vi "TblCheck.vi"(4 "error in":errorcluster, 7 "connection reference":T1) -> (0 "error out":errorcluster, 2 "tables":string[](array[string]), 3 "conn ref out":T1)   [LabVIEW 2010]
uses:
  <vilib>/addons/database/Connection.llb/Conn ObjectReference.ctl
  <vilib>/addons/database/NI_Database_API.lvlib
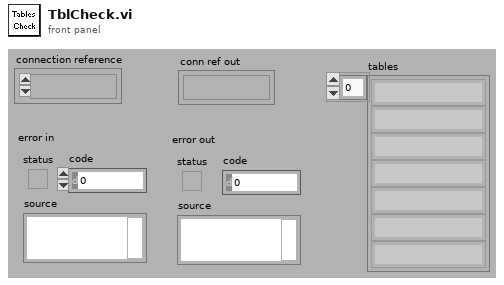
[diagram p1: front panel]
types:
  T1 = typedef "NI_Database_API.lvlib/Conn ObjectReference.ctl" = refnum<k1>
  T2 = cluster{"type":string, "units":string, "n":i32}[]
  T3 = typedef "NI_Database_API.lvlib/DB Tools Column Info.ctl" = cluster{"column name":string, "data type":T4, "size":i32, "allow null?":bool}
  T4 = typedef "NI_Database_API.lvlib/DB Tools DataTypes.ctl" = enum16{"String", "Long (I32)", "Single (SGL)", "Double (DBL)", "Date/Time", "Binary"}
  T5 = cluster{"key":string, "column information":T3[]}[]
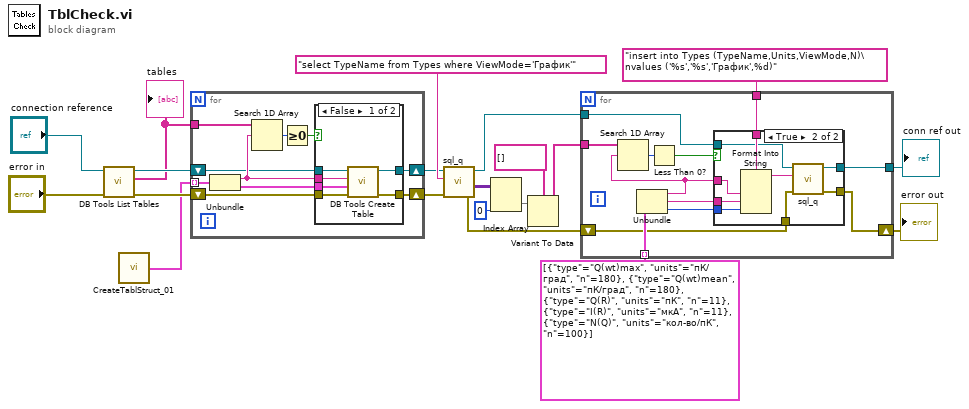
[diagram p0: block diagram]
diagram:
  n1 = call <vilib>:"DB Tools List Tables.vi"("error in (no error)"="error in", "connection reference"="connection reference") -> ("error out"=w19:errorcluster, "tables"=w18:string[], "connection reference out"=w20:T1)  [unwired: 3 in]
  "tables" <- w18
  n2 = call "CreateTablStruct_01.vi"() -> ("Array"=w15:T5)
  n3 = for {
    tunnel: w15 -> [w27] mode=indexing
    tunnel: w18 -> [w30]
    shift-right: [w22] -> w6
    shift-left: w20 -> [w21]
    shift-right: [w24] -> w5
    shift-left: w19 -> [w23]
    n4 = Unbundle(w27) -> ("key"=w26:string, "column information"=w25:T3[])
    n5 = Search 1D Array(1D array=w30, element=w26) -> (index of element=w29:i32)  [unwired: 1 in]
    n6 = Greater Or Equal To 0?(x=w29) -> (x >= 0?=w28:bool)
    n7 = case shown="False" w28 {
      tunnel: w26 -> [w36 _]
      tunnel: w25 -> [w35 _]
      tunnel: [w34 w38] -> w24
      tunnel: w23 -> [w33 w38]
      tunnel: [w32 w37] -> w22
      tunnel: w21 -> [w31 w37]
      frame False {
        n8 = call <vilib>:"DB Tools Create Table.vi"("error in (no error)"=w33, "column information"=w35, "table"=w36, "connection reference"=w31) -> ("error out"=w34:errorcluster, "connection reference out"=w32:T1)  [unwired: 4 in]
      }
      frame True {
      }
    }
  }
  n9 = call "sql_q.vi"("error in"=w5, "SQL query"="select TypeName from Types where ViewMode='График'", "connect ref"=w6) -> ("error out"=w3:errorcluster, "recordset data"=w11:variant[][], "conn ref out"=w4:T1)  [unwired: 1 in, 1 out]
  n10 = Index Array(array=w11, index (col)=0 ("disabled index (col)")) -> (element=w9:variant[])  [unwired: 1 in]
  n11 = Variant To Data(Variant=w9, type=string[] []) -> (data=w7:string[])  [unwired: 1 in, 1 out]
  n12 = for {
    tunnel: "insert into Types (TypeName,Units,ViewMode,N)\nvalues ('%s','%s','График',%d)" -> [w50]
    tunnel: T2 [{"type"="Q(wt)max", "units"="пК/град", "n"=180}, {"type"="Q(wt)mean", "units"="пК/град", "n"=180}, {"type"="Q(R)", "units"="пК", "n"=11}, {"type"="I(R)", "units"="мкА", "n"=11}, {"type"="N(Q)", "units"="кол-во/пК", "n"=100}] -> [w47] mode=indexing
    tunnel: w7 -> [w49]
    tunnel: w4 -> [w42]
    shift-right: [w40] -> w1
    shift-left: w3 -> [w41]
    tunnel: [w39] -> w2
    n13 = Unbundle(w47) -> ("type"=w46:string, "units"=w45:string, "n"=w44:i32)
    n14 = Search 1D Array(1D array=w49, element=w46) -> (index of element=w48:i32)  [unwired: 1 in]
    n15 = Less Than 0?(x=w48) -> (x < 0?=w43:bool)
    n16 = case shown="True" w43 {
      tunnel: w50 -> [_ w61]
      tunnel: w46 -> [_ w59]
      tunnel: w45 -> [_ w58]
      tunnel: w44 -> [_ w57]
      tunnel: w42 -> [w51 w56]
      tunnel: w41 -> [w52 w55]
      tunnel: [w52 w54] -> w40
      tunnel: [w51 w53] -> w39
      frame False {
      }
      frame True {
        n17 = Format Into String(format string=w61, w59, w58, w57) -> (resulting string=w60:string)  [unwired: 2 in, 1 out]
        n18 = call "sql_q.vi"("error in"=w55, "SQL query"=w60, "connect ref"=w56) -> ("error out"=w54:errorcluster, "conn ref out"=w53:T1)  [unwired: 1 in, 2 out]
      }
    }
  }
  "error out" <- w1
  "conn ref out" <- w2
